vi "Set Injected Boolean.vi"(6 "Enable":bool, 8 "error in (no error)":errorcluster, 9 "Value":T1, 10 "Tag":string, 11 "Fault-Injection Bus in":refnum<class "Fault-Injection Bus.lvclass">) -> (0 "error out":errorcluster, 3 "Fault-Injection Bus out":refnum<class "Fault-Injection Bus.lvclass">)   [LabVIEW 2021, in "Fault-Injection Bus.lvclass"]
uses:
  Fault-Injection Bus.lvclass
  Boolean/Support/Value Type.ctl
  Boolean/Fault-Injection_Boolean.lvclass
  C:/Program Files (x86)/National Instruments/LabVIEW 2021/vi.lib/TSA/Abstract Data Classes/Abs_Types/Value/Abs_Value.lvclass
  Fault-Injection Bus.lvclass/Fault-Injection Bus.ctl
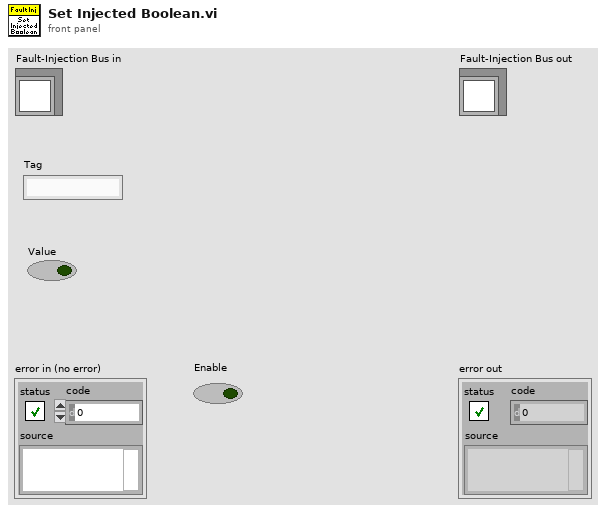
[diagram p1: front panel]
types:
  T1 = typedef "Fault-Injection_Boolean.lvclass/Value Type.ctl" = bool
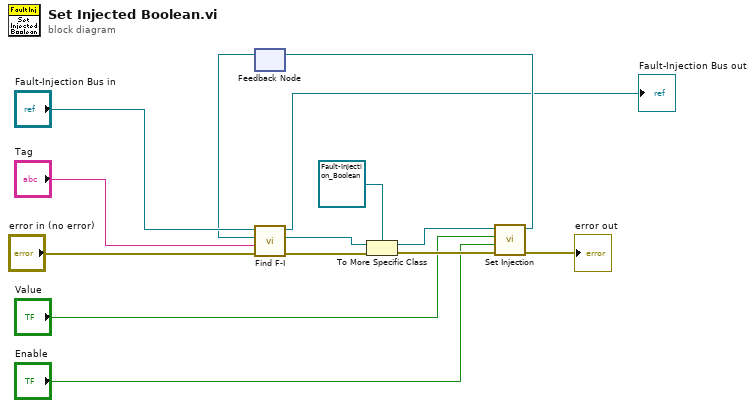
[diagram p0: block diagram]
diagram:
  n1 = feedback #1() -> (w11:refnum<class "Fault-Injection_Boolean.lvclass">)  [unwired: 1 in]
  n2 = call "Find F-I.vi"("error in (no error)"="error in (no error)", "Tag"="Tag", "Abs_Value.lvclass"=w11, "Fault-Injection Bus in"="Fault-Injection Bus in") -> ("error out"=w10:errorcluster, "Abs_Value.lvclass 2"=w9:refnum<class "Abs_Value.lvclass">, "Fault-Injection Bus out"=→"Fault-Injection Bus out":refnum<class "Fault-Injection Bus.lvclass">)  [unwired: 5 in]
  n3 = To More Specific Class(target class=refnum<class "Fault-Injection_Boolean.lvclass"> refnum ("Fault-Injection_Boolean in"), reference=w9, error in=w10) -> (specific class reference=w6:refnum<class "Fault-Injection_Boolean.lvclass">, error out=w7:errorcluster)
  n4 = call "Set Injection.vi"("error in (no error)"=w7, "Enable"="Enable", "Value"="Value", "Fault-Injection_Boolean in"=w6) -> ("error out"=→"error out":errorcluster, "Fault-Injection_Boolean out"=w5:refnum<class "Fault-Injection_Boolean.lvclass">)  [unwired: 6 in]
  n5 = feedback-in #1(w5) -> ()
